vi "Shutdown.vi"(8 "error in":errorcluster, 11 "Power Supply in":refnum<class "Power Supply.lvclass">) -> (0 "error out":errorcluster, 3 "Power Supply out":refnum<class "Power Supply.lvclass">)   [LabVIEW 2018, in "Power Supply.lvlib" / "Power Supply.lvclass"]
doc: "This VI turns off the power supply and closes the resource reference. \n\nIt bypasses error inputs to force safe shutdown."
uses:
  Power Supply.lvclass
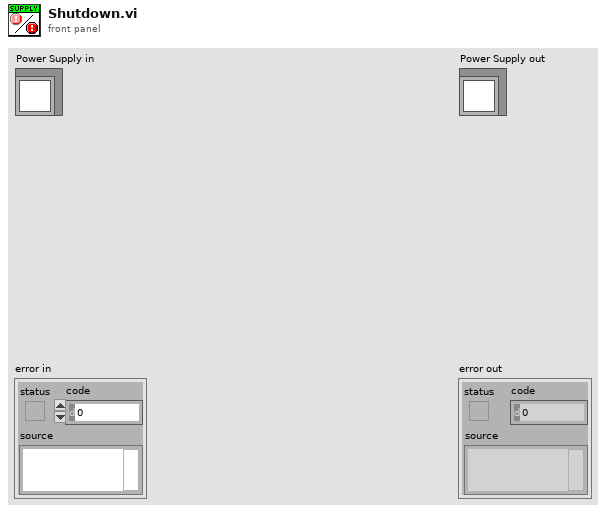
[diagram p1: front panel]
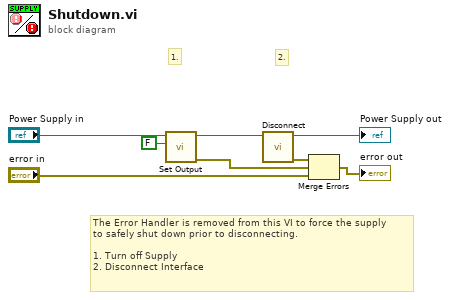
[diagram p0: block diagram]
diagram:
  # "2."
  # "1."
  # "The Error Handler is removed from this VI to force the supply\nto safely shut down prior to disconnecting.\n\n1. Turn off Supply\n2. Disconnect Interface"
  n1 = call "Set Output.vi"("Output"=FALSE, "Power Supply in"="Power Supply in") -> ("error out"=w3:errorcluster, "Power Supply out"=w6:refnum<class "Power Supply.lvclass">)  [unwired: 8 in]
  n2 = call-dynamic "Disconnect.vi"("Power Supply in"=w6) -> ("error out"=w4:errorcluster, "Power Supply out"=→"Power Supply out":refnum<class "Power Supply.lvclass">)  [unwired: 9 in]
  n3 = Merge Errors(w4, w3, "error in") -> (→"error out":errorcluster)
